vi "Calc_Moment.vi"(8 "Center State at T":T2, 9 "Initial Anchor Position":dbl[][](array[numeric]), 10 "Extention":dbl[][](array[numeric]), 11 "On_Particle State":T1(array[cluster])) -> (0 "Center State at T 2":T2, 2 "SummedMoment":dbl, 3 "On_Particle State":T1(array[cluster]))   [LabVIEW 2020]
uses:
  <vilib>/Analysis/baseanly.llb/Mean (DBL).vi
  <vilib>/Analysis/baseanly.llb/Real Outer Product.vi
  <vilib>/Analysis/NI_AALBase.lvlib
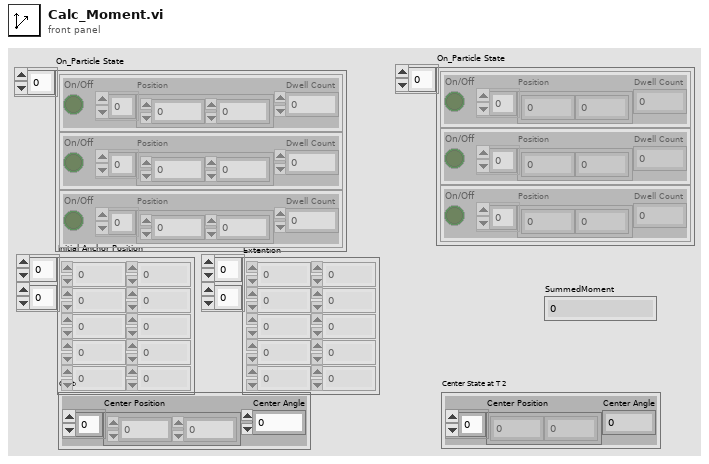
[diagram p1: front panel]
types:
  T1 = cluster{"On/Off":bool, "Position":dbl[], "Dwell Count":i32}[]
  T2 = cluster{"Center Position":dbl[], "Center Angle":dbl}
  T3 = typedef "NI_Matrix.lvlib/RealMatrix.ctl" = dbl[][]
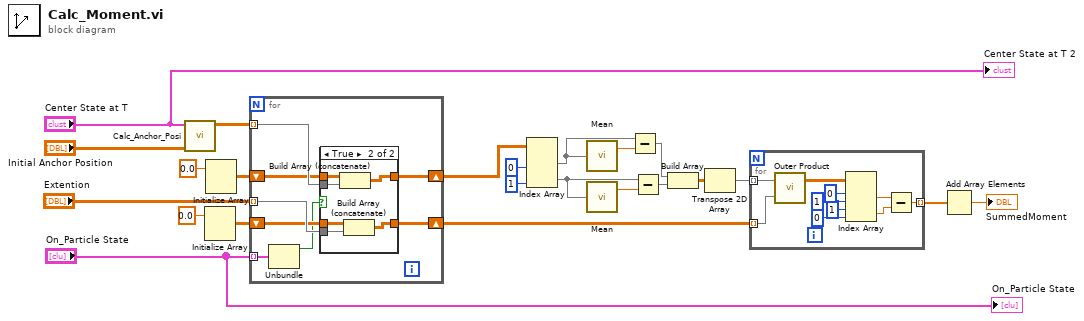
[diagram p0: block diagram]
diagram:
  n1 = call "Calc_Anchor_Posi.vi"("Initial Anchor Position"="Initial Anchor Position", "Center State at T"="Center State at T") -> ("Anchor Posi at T"=w9:dbl[][])  [unwired: 9 in]
  n2 = Initialize Array(0.0 ("element")) -> (w6:dbl[][])  [unwired: 2 in]
  n3 = Initialize Array(0.0 ("element")) -> (w4:dbl[][])  [unwired: 2 in]
  n4 = for {
    tunnel: w9 -> [w31] mode=indexing
    tunnel: "Extention" -> [w30] mode=indexing
    shift-right: [w26] -> w2
    shift-left: w6 -> [w29]
    shift-right: [w27] -> w3
    shift-left: w4 -> [w28]
    tunnel: "On_Particle State" -> [w25] mode=indexing
    n5 = Unbundle(w25) -> ("On/Off"=w24:bool)  [unwired: 2 out]
    n6 = case shown="TRUE" w24 {
      tunnel: w31 -> [_ w39]
      tunnel: w30 -> [_ w38]
      tunnel: w29 -> [w32 w37]
      tunnel: w28 -> [w33 w36]
      tunnel: [w33 w35] -> w27
      tunnel: [w32 w34] -> w26
      frame False {
      }
      frame True {
        n7 = Build Array (concatenate)(w36, w39) -> (w35:dbl[][])
        n8 = Build Array (concatenate)(w37, w38) -> (w34:dbl[][])
      }
    }
  }
  n9 = Index Array(array=w3, index (col) #1=0 ("index (row)"), index (col) #2=1 ("index (row)")) -> (element #1=w17:dbl[], element #2=w16:dbl[])  [unwired: 2 in]
  n10 = call-poly <vilib>:"Mean.vi"("X"=w17) -> ("mean"=w13:dbl)  [unwired: 1 out]
  n11 = call-poly <vilib>:"Mean.vi"("X"=w16) -> ("mean"=w12:dbl)  [unwired: 1 out]
  n12 = Subtract(x=w17, y=w13) -> (x-y=w21:dbl[])
  n13 = Subtract(x=w16, y=w12) -> (x-y=w20:dbl[])
  n14 = Build Array(w21, w20) -> (w23:dbl[][])
  n15 = Transpose 2D Array(2D array=w23) -> (transposed array=w22:dbl[][])
  n16 = for {
    tunnel: w22 -> [w49] mode=indexing
    tunnel: w2 -> [w48] mode=indexing
    tunnel: [w42] -> w19 mode=indexing
    n17 = call-poly <vilib>:"Outer Product.vi"("Y Vector"=w48, "X Vector"=w49) -> ("Outer Product"=w41:T3)  [unwired: 1 out]
    n18 = Index Array(array=w41, index (row) #1=0 ("index (row)"), index (col) #1=1 ("disabled index (col)"), index (row) #2=1 ("index (row)"), index (col) #2=0 ("disabled index (col)")) -> (element #1=w43:dbl, element #2=w40:dbl)
    n19 = Subtract(x=w43, y=w40) -> (x-y=w42:dbl)
  }
  n20 = Add Array Elements(numeric array=w19) -> (sum=→"SummedMoment":dbl)
  "Center State at T 2" <- "Center State at T"
  "On_Particle State" <- "On_Particle State"
